vi "SaveData.vi"(8 "에러 입력":errorcluster, 9 "Index":i32, 10 "배열":T1(array[cluster]), 11 "참조번호":refnum<file>) -> (0 "에러 출력":errorcluster, 1 "Index 2":i32, 3 "참조 번호 출력":refnum<file>)   [LabVIEW 2019]
types:
  T1 = cluster{"Q_motor":cluster{"Actual Pos_0":i32, "Actual Vel_0":i32, "Target Cur_0":i32, "Actual Cur_0":i32, "Actual Pos_1":i32, "Actual Vel_1":i32, "Target Cur_1":i32, "Actual Cur_1":i32, "status_0 ":u16, "status_1":u16}, "Q_PSDtoSAVE":i32, "Q_MOTORtoSAVE":i32, "Save_Loop time":dbl, "Save_Integrated time":dbl, "Process":cluster{"Status_PS":string, "Q to xsensor":bool, "FPGA_data":sgl[], "R_force":sgl, "L_force":sgl, "Param":cluster{"Init_Onset_Load":sgl, "Pos_base_L":sgl, "Pos_base_R":sgl, "Init_Vel":i32, "Init_Accel":u32, "Test_Vel":i32, "Test_Acc":u32, "Load_Warning":sgl, "Load_Alarm":sgl, "Control param In":cluster{"L_velocity":u32, "L_Power":sgl, "R_velocity":u32, "R_Power":sgl, "T_param_L":cluster{"Onset":sgl, "Peak":sgl, "End":sgl, "검출값":sgl, "기준값":sgl}, "T_param_R":cluster{"Onset":sgl, "Peak":sgl, "Release":sgl, "검출값":sgl, "기준값":sgl}, "Initialize?":bool, "CAN read?":bool, "Optimal count":i32, "Velocity range":cluster{"Output high":dbl, "Output low":dbl}}, "Init_R":bool, "Init_L":bool, "Force_mode_R":bool, "Force mode_L":bool, "GCP_L":sgl, "GCP_R":sgl, "D_Vel_L":sgl, "D_Vel_R":sgl, "D_Cur_L(/1000)":sgl, "D_Cur_R(/1000)":sgl, "Force_reference_L":sgl, "Force_reference_R":sgl, "Initial_IMU_L":sgl, "Initial_IMU_R":sgl, "L_NUM":u32, "L_Period":i16, "R_NUM":u32, "R_Period":i16, "Initialization count":i32, "R_Ctrl_St":bool, "L_Ctrl_St":bool}}, "GCP":cluster{"R_angvel_raw":sgl, "R_angvel_filt":sgl, "L_angvel_raw":sgl, "L_angvel_filt":sgl, "Q_GCP":cluster{"L_num":u32, "L_GCP":dbl, "L_Period":u32, "R_num":u32, "R_GCP":dbl, "R_Period":u32, "L_Ctrl_St":bool, "R_Ctrl_St":bool}}, "Q_GCPtoSAVE":i32, "Save_loop":i64}[]
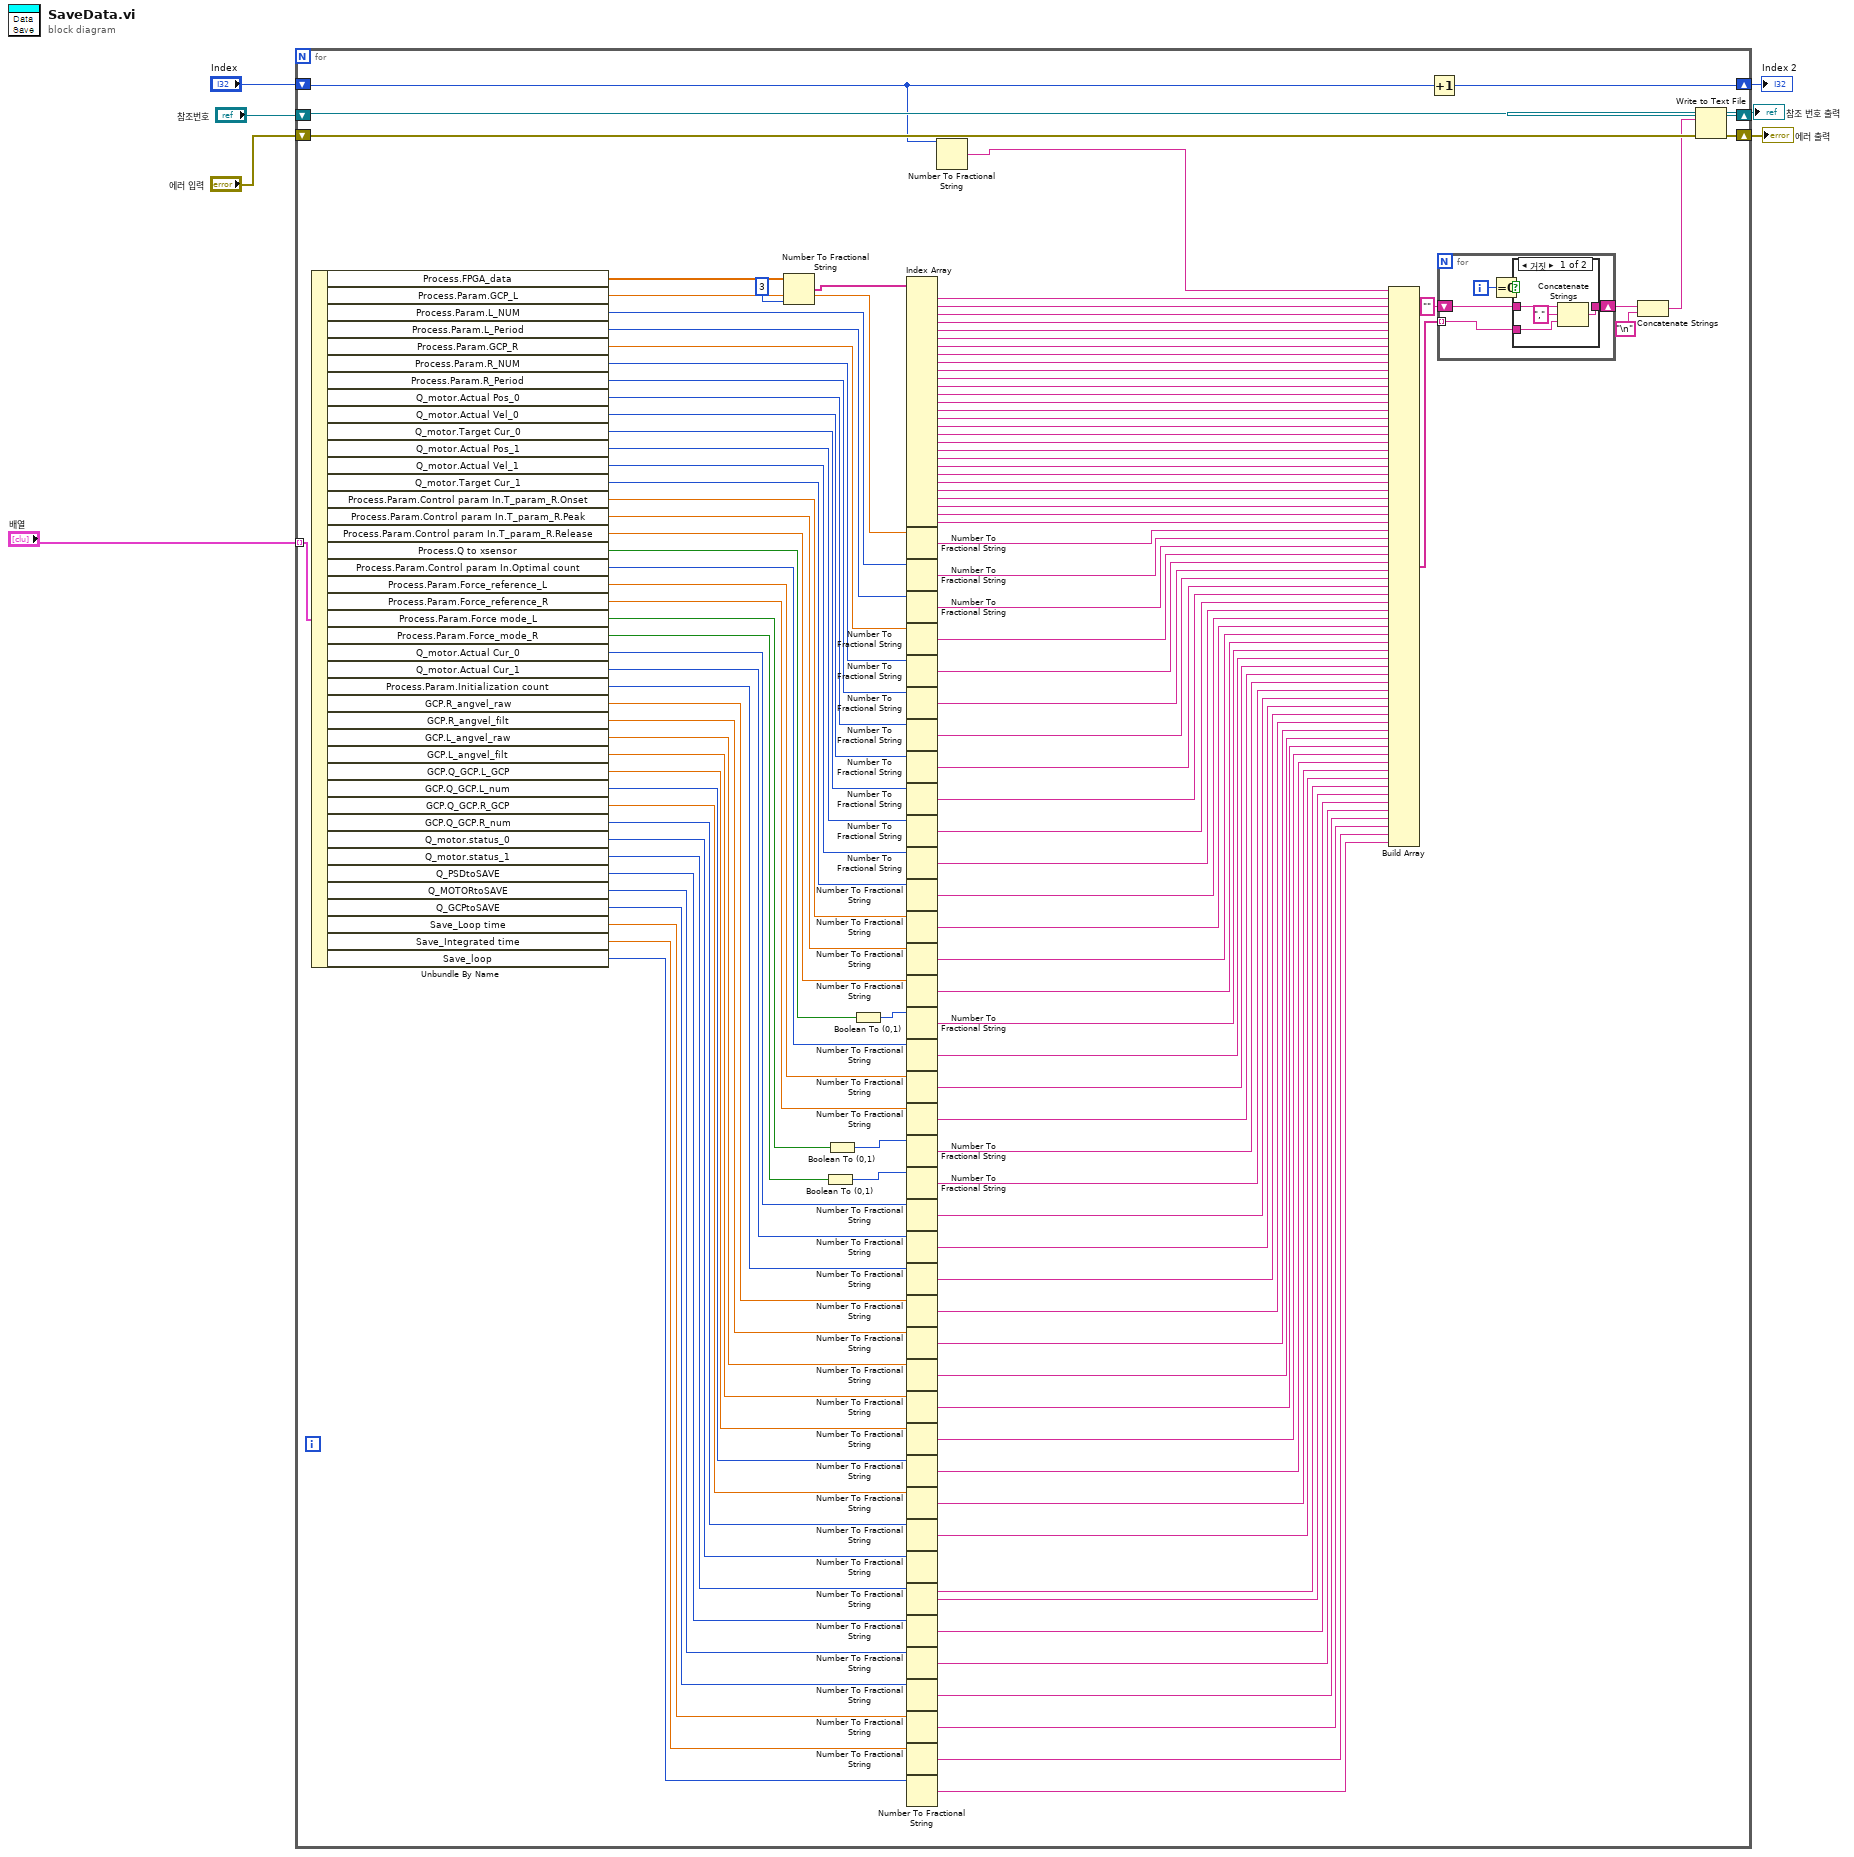
[diagram p0: block diagram]
diagram:
  n1 = for {
    shift-right: [w133] -> w4
    shift-left: "에러 입력" -> [w135]
    shift-right: [w134] -> w5
    shift-left: "참조번호" -> [w109]
    shift-right: [w103] -> w2
    shift-left: "Index" -> [w41]
    tunnel: "배열" -> [w102] mode=indexing
    n2 = Unbundle By Name(w102) -> ("Process.FPGA_data"=w131:sgl[], "Process.Param.GCP_L"=w92:sgl, "Process.Param.L_NUM"=w91:u32, "Process.Param.L_Period"=w90:i16, "Process.Param.GCP_R"=w89:sgl, "Process.Param.R_NUM"=w88:u32, "Process.Param.R_Period"=w87:i16, "Q_motor.Actual Pos_0"=w86:i32, "Q_motor.Actual Vel_0"=w85:i32, "Q_motor.Target Cur_0"=w84:i32, "Q_motor.Actual Pos_1"=w83:i32, "Q_motor.Actual Vel_1"=w82:i32, "Q_motor.Target Cur_1"=w81:i32, "Process.Param.Control param In.T_param_R.Onset"=w66:sgl, "Process.Param.Control param In.T_param_R.Peak"=w65:sgl, "Process.Param.Control param In.T_param_R.Release"=w60:sgl, "Process.Q to xsensor"=w64:bool, "Process.Param.Control param In.Optimal count"=w61:i32, "Process.Param.Force_reference_L"=w55:sgl, "Process.Param.Force_reference_R"=w54:sgl, "Process.Param.Force mode_L"=w53:bool, "Process.Param.Force_mode_R"=w52:bool, "Q_motor.Actual Cur_0"=w46:i32, "Q_motor.Actual Cur_1"=w47:i32, "Process.Param.Initialization count"=w43:i32, "GCP.R_angvel_raw"=w39:sgl, "GCP.R_angvel_filt"=w38:sgl, "GCP.L_angvel_raw"=w23:sgl, "GCP.L_angvel_filt"=w22:sgl, "GCP.Q_GCP.L_GCP"=w18:dbl, "GCP.Q_GCP.L_num"=w21:u32, "GCP.Q_GCP.R_GCP"=w20:dbl, "GCP.Q_GCP.R_num"=w19:u32, "Q_motor.status_0"=w35:u16, "Q_motor.status_1"=w34:u16, "Q_PSDtoSAVE"=w31:i32, "Q_MOTORtoSAVE"=w30:i32, "Q_GCPtoSAVE"=w17:i32, "Save_Loop time"=w29:dbl, "Save_Integrated time"=w28:dbl, "Save_loop"=w9:i64)
    n3 = Number To Fractional String(number=w131, precision (6)=i16 3 ("정밀도(6)")) -> (F-format string=w130:string[])  [unwired: 2 in]
    n4 = Boolean To (0,1)(Boolean=w52) -> (0, 1=w56:i16)
    n5 = Boolean To (0,1)(Boolean=w53) -> (0, 1=w57:i16)
    n6 = Boolean To (0,1)(Boolean=w64) -> (0, 1=w63:i16)
    n7 = Index Array(array=w130) -> (element #1=w129:string, element #2=w128:string, element #3=w127:string, element #4=w126:string, element #5=w125:string, element #6=w124:string, element #7=w123:string, element #8=w122:string, element #9=w121:string, element #10=w120:string, element #11=w119:string, element #12=w118:string, element #13=w117:string, element #14=w116:string, element #15=w115:string, element #16=w114:string, element #17=w113:string, element #18=w112:string, element #19=w111:string, element #20=w110:string, element #21=w101:string, element #22=w100:string, element #23=w99:string, element #24=w98:string, element #25=w97:string, element #26=w96:string, element #27=w95:string, element #28=w94:string, element #29=w93:string)  [unwired: 29 in]
    n8 = Number To Fractional String(number=w92) -> (F-format string=w80:string)  [unwired: 3 in]
    n9 = Number To Fractional String(number=w91) -> (F-format string=w79:string)  [unwired: 3 in]
    n10 = Number To Fractional String(number=w90) -> (F-format string=w78:string)  [unwired: 3 in]
    n11 = Number To Fractional String(number=w89) -> (F-format string=w77:string)  [unwired: 3 in]
    n12 = Number To Fractional String(number=w88) -> (F-format string=w76:string)  [unwired: 3 in]
    n13 = Number To Fractional String(number=w87) -> (F-format string=w75:string)  [unwired: 3 in]
    n14 = Number To Fractional String(number=w86) -> (F-format string=w74:string)  [unwired: 3 in]
    n15 = Number To Fractional String(number=w85) -> (F-format string=w73:string)  [unwired: 3 in]
    n16 = Number To Fractional String(number=w84) -> (F-format string=w72:string)  [unwired: 3 in]
    n17 = Number To Fractional String(number=w83) -> (F-format string=w71:string)  [unwired: 3 in]
    n18 = Number To Fractional String(number=w82) -> (F-format string=w70:string)  [unwired: 3 in]
    n19 = Number To Fractional String(number=w81) -> (F-format string=w69:string)  [unwired: 3 in]
    n20 = Number To Fractional String(number=w66) -> (F-format string=w68:string)  [unwired: 3 in]
    n21 = Number To Fractional String(number=w65) -> (F-format string=w67:string)  [unwired: 3 in]
    n22 = Number To Fractional String(number=w60) -> (F-format string=w58:string)  [unwired: 3 in]
    n23 = Number To Fractional String(number=w63) -> (F-format string=w62:string)  [unwired: 3 in]
    n24 = Number To Fractional String(number=w61) -> (F-format string=w59:string)  [unwired: 3 in]
    n25 = Number To Fractional String(number=w55) -> (F-format string=w51:string)  [unwired: 3 in]
    n26 = Number To Fractional String(number=w54) -> (F-format string=w50:string)  [unwired: 3 in]
    n27 = Number To Fractional String(number=w57) -> (F-format string=w49:string)  [unwired: 3 in]
    n28 = Number To Fractional String(number=w56) -> (F-format string=w48:string)  [unwired: 3 in]
    n29 = Number To Fractional String(number=w46) -> (F-format string=w44:string)  [unwired: 3 in]
    n30 = Number To Fractional String(number=w47) -> (F-format string=w45:string)  [unwired: 3 in]
    n31 = Number To Fractional String(number=w43) -> (F-format string=w42:string)  [unwired: 3 in]
    n32 = Number To Fractional String(number=w39) -> (F-format string=w37:string)  [unwired: 3 in]
    n33 = Number To Fractional String(number=w38) -> (F-format string=w36:string)  [unwired: 3 in]
    n34 = Number To Fractional String(number=w23) -> (F-format string=w16:string)  [unwired: 3 in]
    n35 = Number To Fractional String(number=w22) -> (F-format string=w15:string)  [unwired: 3 in]
    n36 = Number To Fractional String(number=w18) -> (F-format string=w14:string)  [unwired: 3 in]
    n37 = Number To Fractional String(number=w21) -> (F-format string=w13:string)  [unwired: 3 in]
    n38 = Number To Fractional String(number=w20) -> (F-format string=w12:string)  [unwired: 3 in]
    n39 = Number To Fractional String(number=w19) -> (F-format string=w11:string)  [unwired: 3 in]
    n40 = Number To Fractional String(number=w35) -> (F-format string=w33:string)  [unwired: 3 in]
    n41 = Number To Fractional String(number=w34) -> (F-format string=w32:string)  [unwired: 3 in]
    n42 = Number To Fractional String(number=w31) -> (F-format string=w27:string)  [unwired: 3 in]
    n43 = Number To Fractional String(number=w30) -> (F-format string=w26:string)  [unwired: 3 in]
    n44 = Number To Fractional String(number=w17) -> (F-format string=w10:string)  [unwired: 3 in]
    n45 = Number To Fractional String(number=w29) -> (F-format string=w25:string)  [unwired: 3 in]
    n46 = Number To Fractional String(number=w28) -> (F-format string=w24:string)  [unwired: 3 in]
    n47 = Number To Fractional String(number=w9) -> (F-format string=w8:string)  [unwired: 3 in]
    n48 = Number To Fractional String(number=w41) -> (F-format string=w40:string)  [unwired: 3 in]
    n49 = Build Array(w40, w129, w128, w127, w126, w125, w124, w123, w122, w121, w120, w119, w118, w117, w116, w115, w114, w113, w112, w111, w110, w101, w100, w99, w98, w97, w96, w95, w94, w93, w80, w79, w78, w77, w76, w75, w74, w73, w72, w71, w70, w69, w68, w67, w58, w62, w59, w51, w50, w49, w48, w44, w45, w42, w37, w36, w16, w15, w14, w13, w12, w11, w33, w32, w27, w26, w10, w25, w24, w8) -> (w105:string[])
    n50 = Increment(x=w41) -> (x+1=w103:i32)
    n51 = for {
      shift-right: [w137] -> w107
      shift-left: "" -> [w138]
      tunnel: w105 -> [w136] mode=indexing
      i -> [w140]
      n52 = Equal To 0?(x=w140) -> (x = 0?=w139:bool)
      n53 = case shown="거짓" w139 {
        tunnel: w138 -> [w144 w145]
        tunnel: [w143 w145] -> w137
        tunnel: w136 -> [w141 _]
        frame False {
          n54 = Concatenate Strings(w144, "," ("문자열"), w141) -> (w143:string)
        }
        frame True {
        }
      }
    }
    n55 = Concatenate Strings(w107, "\n") -> (w108:string)
    n56 = Write to Text File(file (use dialog)=w109, text=w108, error in=w135) -> (refnum out=w134:refnum<file>, error out=w133:errorcluster)  [unwired: 1 in, 1 out]
  }
  "참조 번호 출력" <- w5
  "에러 출력" <- w4
  "Index 2" <- w2
